vi "Config - DTO round trip.vi"(8 "error in (no error)":errorcluster) -> (0 "error out":errorcluster)   [LabVIEW 2026, in "Tests.lvlib"]
doc: "Unit test (Caraya): verifies a configuration survives a round trip through its JSON DTO representation and back unchanged (SRS-050a).\nMaps a populated native config to its DTO mirror and back, then asserts the round-tripped config equals the original, so serialization and the field mappings introduce no drift.\nTests.lvlib, friend of Lumberjack.lvlib; unit tier.\n\nImplements LMBR-T-061 -> SRS-050a. Assert-level IDs: Test-ID-Assert-Checklist.md.\n\nImplements LMBR-T-061 -> SRS-050a. Assert-level IDs: Test-ID-Assert-Checklist.md."
uses:
  Tests.lvlib
  src/TypeDefs/ConfigDTO/AppenderConfigDTO.ctl
  src/TypeDefs/ConfigDTO/FilterDTO.ctl
  src/TypeDefs/ConfigDTO/FileAppenderConfigDTO.ctl
  src/TypeDefs/ConfigDTO/FileConfigDTO.ctl
  src/TypeDefs/ConfigDTO/LumberjackConfigDTO.ctl
  <vilib>/addons/_JKI Toolkits/Caraya/classes/Assert/Assert Equal Value_Variant.vi
  <vilib>/addons/_JKI Toolkits/Caraya/classes/Test/Test.lvclass
  src/Lumberjack.lvlib
  <vilib>/addons/_JKI Toolkits/Caraya/classes/Assert/Assert.lvclass
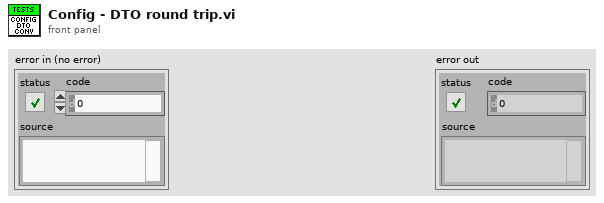
[diagram p1: front panel]
types:
  T1 = typedef "Lumberjack.lvlib/FileConfigDTO.ctl" = cluster{"rootFolder":string, "maxFileSize":i64, "maxFileCount":i32, "baseName":string, "extension":string, "delimiter":string, "calendarFolderTree":bool}
  T2 = typedef "Lumberjack.lvlib/LumberjackConfigDTO.ctl" = cluster{"schemaVersion":string, "globalThreshold":string, "defaultFileAppender":T3}
  T3 = typedef "Lumberjack.lvlib/FileAppenderConfigDTO.ctl" = cluster{"common":T4, "file":T1}
  T4 = typedef "Lumberjack.lvlib/AppenderConfigDTO.ctl" = cluster{"id":string, "threshold":string, "filter":T5, "queueBound":i32, "dropPolicy":string, "useUTC":bool}
  T5 = typedef "Lumberjack.lvlib/FilterDTO.ctl" = cluster{"mode":string, "levelMin":string, "levelMax":string, "tagPrefix":string}
  T6 = typedef "Lumberjack.lvlib/Filter.ctl" = cluster{"mode":T7, "levelMin":T8, "levelMax":T8, "tagPrefix":string}
  T7 = typedef "Lumberjack.lvlib/FilterMode.ctl" = enum16{"Mirror", "Routed"}
  T8 = typedef "Lumberjack.lvlib/Severity.ctl" = enum16{"OFF", "FATAL", "ERROR", "WARN", "INFO", "DEBUG", "TRACE", "ALL"}
  T9 = typedef "Lumberjack.lvlib/AppenderConfig.ctl" = cluster{"id":string, "threshold":T8, "filter":T6, "queueBound":i32, "dropPolicy":T10, "useUTC":bool}
  T10 = typedef "Lumberjack.lvlib/DropPolicy.ctl" = enum16{"DropOldest", "DropNewest", "LevelAware"}
  T11 = typedef "Lumberjack.lvlib/FileConfig.ctl" = cluster{"rootFolder":path, "maxFileSize":i64, "maxFileCount":i32, "baseName":string, "extension":string, "delimiter":string, "calendarFolderTree":bool}
  T12 = typedef "Lumberjack.lvlib/FileAppenderConfig.ctl" = cluster{"common":T9, "file":T11}
  T13 = typedef "Lumberjack.lvlib/LumberjackConfig.ctl" = cluster{"schemaVersion":string, "globalThreshold":T8, "defaultFileAppender":T12}
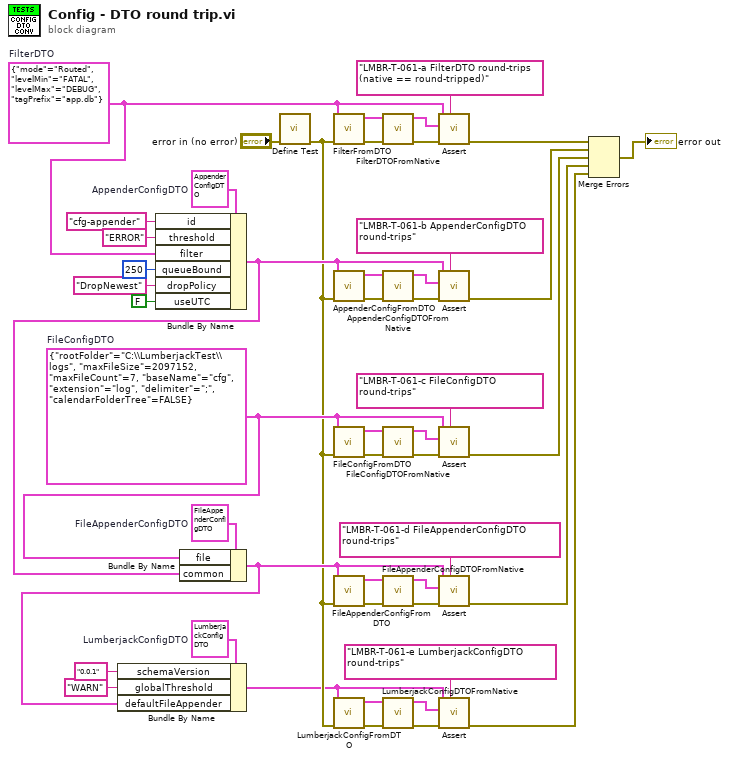
[diagram p0: block diagram]
diagram:
  w20 = T1 {"rootFolder"="C:\\LumberjackTest\\logs", "maxFileSize"=2097152, "maxFileCount"=7, "baseName"="cfg", "extension"="log", "delimiter"=";", "calendarFolderTree"=FALSE}  # FileConfigDTO
  w36 = T2 {"schemaVersion"="", "globalThreshold"="INFO", "defaultFileAppender"={"common"={"id"="", "threshold"="INFO", "filter"={"mode"="mirror", "levelMin"="INFO", "levelMax"="INFO", "tagPrefix"=""}, "queueBound"=0, "dropPolicy"="dropOldest", "useUTC"=FALSE}, "file"={"rootFolder"="", "maxFileSize"=0, "maxFileCount"=0, "baseName"="", "extension"="", "delimiter"="", "calendarFolderTree"=FALSE}}}  # LumberjackConfigDTO
  w23 = T5 {"mode"="Routed", "levelMin"="FATAL", "levelMax"="DEBUG", "tagPrefix"="app.db"}  # FilterDTO
  w32 = T3 {"common"={"id"="", "threshold"="INFO", "filter"={"mode"="Mirror", "levelMin"="INFO", "levelMax"="INFO", "tagPrefix"=""}, "queueBound"=0, "dropPolicy"="DropOldest", "useUTC"=FALSE}, "file"={"rootFolder"="", "maxFileSize"=0, "maxFileCount"=0, "baseName"="", "extension"="", "delimiter"="", "calendarFolderTree"=FALSE}}  # FileAppenderConfigDTO
  w33 = T4 {"id"="", "threshold"="INFO", "filter"={"mode"="Mirror", "levelMin"="INFO", "levelMax"="INFO", "tagPrefix"=""}, "queueBound"=0, "dropPolicy"="DropOldest", "useUTC"=FALSE}  # AppenderConfigDTO
  n1 = Bundle By Name(cluster=w33, "id"="cfg-appender", "threshold"="ERROR", "filter"=w23, "queueBound"=250, "dropPolicy"="DropNewest", "useUTC"=FALSE) -> (w22:T4)
  n2 = Bundle By Name(cluster=w32, "file"=w20, "common"=w22) -> (w18:T3)
  n3 = Bundle By Name(cluster=w36, "schemaVersion"="0.0.1", "globalThreshold"="WARN", "defaultFileAppender"=w18) -> (w15:T2)
  n4 = call <vilib>:"Define Test.vi"("error in (no error)"="error in (no error)") -> ("error out"=w17:errorcluster)  [unwired: 9 in, 1 out]
  n5 = call "FilterFromDTO.vi"("error in (no error)"=w17, "FilterDTO"=w23) -> ("error out"=w43:errorcluster, "Filter"=w44:T6)  [unwired: 8 in]
  n6 = call "AppenderConfigFromDTO.vi"("error in (no error)"=w17, "AppenderConfigDTO"=w22) -> ("error out"=w37:errorcluster, "AppenderConfig"=w38:T9)  [unwired: 8 in]
  n7 = call "FileConfigFromDTO.vi"("error in (no error)"=w17, "FileConfigDTO"=w20) -> ("error out"=w41:errorcluster, "FileConfig"=w42:T11)  [unwired: 8 in]
  n8 = call "FileAppenderConfigFromDTO.vi"("error in (no error)"=w17, "FileAppenderConfigDTO"=w18) -> ("error out"=w39:errorcluster, "FileAppenderConfig"=w40:T12)  [unwired: 8 in]
  n9 = call "LumberjackConfigFromDTO.vi"("error in (no error)"=w17, "LumberjackConfigDTO"=w15) -> ("error out"=w45:errorcluster, "LumberjackConfig"=w46:T13)  [unwired: 8 in]
  n10 = call "FilterDTOFromNative.vi"("error in (no error)"=w43, "Filter"=w44) -> ("error out"=w26:errorcluster, "FilterDTO"=w25:T5)  [unwired: 8 in]
  n11 = call "AppenderConfigDTOFromNative.vi"("error in (no error)"=w37, "AppenderConfig"=w38) -> ("error out"=w24:errorcluster, "AppenderConfigDTO"=w14:T4)  [unwired: 8 in]
  n12 = call "FileConfigDTOFromNative.vi"("error in (no error)"=w41, "FileConfig"=w42) -> ("error out"=w21:errorcluster, "FileConfigDTO"=w13:T1)  [unwired: 8 in]
  n13 = call "FileAppenderConfigDTOFromNative.vi"("error in (no error)"=w39, "FileAppenderConfig"=w40) -> ("error out"=w19:errorcluster, "FileAppenderConfigDTO"=w12:T3)  [unwired: 8 in]
  n14 = call "LumberjackConfigDTOFromNative.vi"("error in (no error)"=w45, "LumberjackConfig"=w46) -> ("error out"=w16:errorcluster, "LumberjackConfigDTO"=w11:T2)  [unwired: 8 in]
  n15 = call-poly <vilib>:"Assert.vi"("Label"="LMBR-T-061-a FilterDTO round-trips (native == round-tripped)", "error in (no error)"=w26, "Actual"=w25, "Expected"=w23) -> ("error out"=w10:errorcluster)  [unwired: 6 in, 1 out]
  n16 = call-poly <vilib>:"Assert.vi"("Label"="LMBR-T-061-b AppenderConfigDTO round-trips", "error in (no error)"=w24, "Actual"=w14, "Expected"=w22) -> ("error out"=w9:errorcluster)  [unwired: 6 in, 1 out]
  n17 = call-poly <vilib>:"Assert.vi"("Label"="LMBR-T-061-c FileConfigDTO round-trips", "error in (no error)"=w21, "Actual"=w13, "Expected"=w20) -> ("error out"=w8:errorcluster)  [unwired: 6 in, 1 out]
  n18 = call-poly <vilib>:"Assert.vi"("Label"="LMBR-T-061-d FileAppenderConfigDTO round-trips", "error in (no error)"=w19, "Actual"=w12, "Expected"=w18) -> ("error out"=w7:errorcluster)  [unwired: 6 in, 1 out]
  n19 = call-poly <vilib>:"Assert.vi"("Label"="LMBR-T-061-e LumberjackConfigDTO round-trips", "error in (no error)"=w16, "Actual"=w11, "Expected"=w15) -> ("error out"=w6:errorcluster)  [unwired: 6 in, 1 out]
  n20 = Merge Errors(w10, w9, w8, w7, w6) -> (→"error out":errorcluster)
